vi "HP 6643A - GPIB Control.vi"() -> ()   [LabVIEW 2018]
doc: "This example performs a serial port write and a serial port read. The parameters set for the serial port must match the parameters of the connected instrument or device. The VISA Configure Serial Port VI sets the configuration parameters. The front panel displays the controls used to configure the basic parameters, such as baud rate, data bits, and parity. The VI passes the VISA resource name to other VIs that perform operations on that VISA resource. The VISA Write function sends a command to the serial device and the VISA Read function returns data based on the command. The VISA Close function then closes the reference to the serial device. It is important to close the reference; otherwise, further communication through that port might not be possible."
uses:
  <vilib>/Instr/_visa.llb/VISA Open Access Mode.ctl
panel:
  in  "Numeric":sgl format="%#.3f"
  out "Current (Amps)":dbl format="%.2f"
  out "Voltage (Volts)":dbl format="%.2f"
  in  "Output":bool
  out "Iterations":i32
  in  "stop":bool
  out "NewVal":dbl
  out "OldVal":dbl
  out "String":string
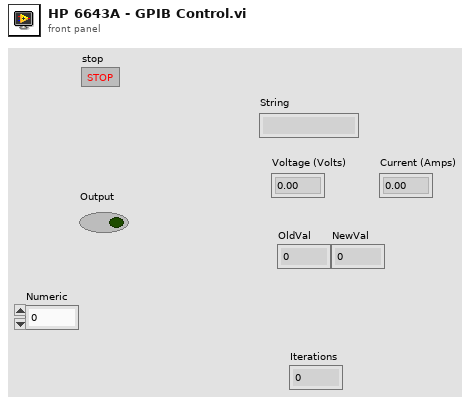
[diagram p1: front panel]
types:
  T1 = typedef "VISA Open Access Mode.ctl" = u32
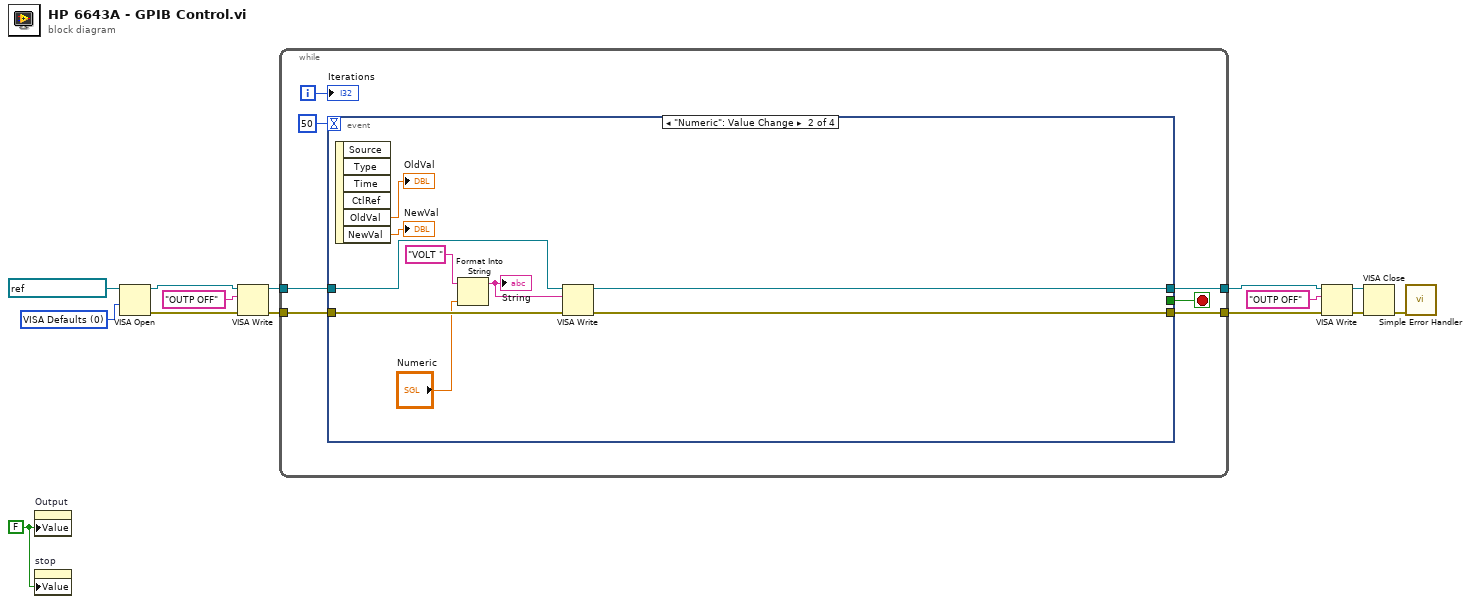
[diagram p0: block diagram]
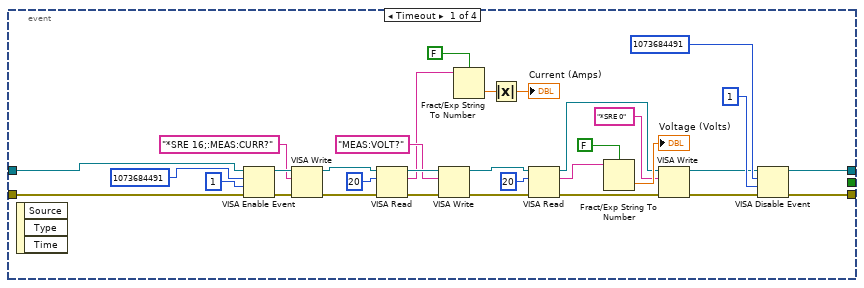
[diagram p2: hidden frame]
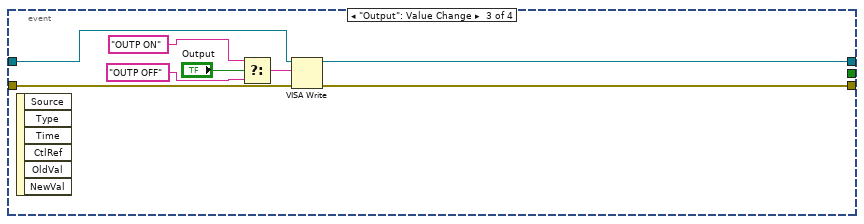
[diagram p3: hidden frame]
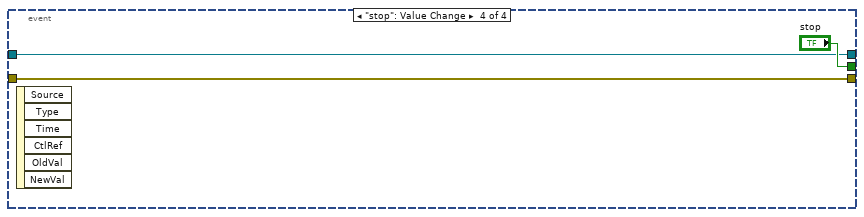
[diagram p4: hidden frame]
diagram:
  w2 = FALSE ("stop")
  w13 = T1 0 items=["VISA Defaults"=0, "Exclusive Lock"=1, "Load Configured Settings"=4] ("Access Mode")
  n1 = property on="Output" class="Bool (strict)"("Value"=w2) -> ()  [unwired: 2 in, 2 out]
  n2 = property on="stop" class="Bool (strict)"("Value"=w2) -> ()  [unwired: 2 in, 2 out]
  n3 = VISA Open(access mode=w13, VISA resource name=refnum<visa-resource-name> "DESK-06643A") -> (VISA resource name=w6:refnum<visa-resource-name>, error out=w7:errorcluster)  [unwired: 3 in]
  n4 = VISA Write(VISA resource name=w6, write buffer="OUTP OFF", error in (no error)=w7) -> (VISA resource name out=w4:refnum<visa-resource-name>, error out=w3:errorcluster)  [unwired: 1 out]
  n5 = while {
    tunnel: w3 -> [w21]
    tunnel: w4 -> [w20]
    tunnel: [w18] -> w10
    tunnel: [w19] -> w12
    i -> [w16]
    stop <- w17 stop-if-true
    n6 = event shown="[1] \"Numeric\": Value Change" {
      selector: _ -> [_ _ _ _]
      dyn-events: _ -> [_ _ _ _]
      timeout: 50 -> [_ _ _ _]
      tunnel: w21 -> [w25 w59 w69 w71]
      tunnel: w20 -> [w26 w60 w70 w72]
      tunnel: [w23 w58 w68 w71] -> w19
      tunnel: [w24 w57 w67 w72] -> w18
      tunnel: [_ _ _ "stop"] -> w17
      event Timeout {
        n7 = event-data() -> ()  [unwired: 1 in, 3 out]
        n8 = VISA Enable Event(8:w25, 9:u16 1, 10:u32 1073684491, 11:w26) -> (0:w38:errorcluster, 3:w39:refnum<visa-resource-name>)
        n9 = VISA Write(VISA resource name=w39, write buffer="*SRE 16;:MEAS:CURR?", error in (no error)=w38) -> (VISA resource name out=w30:refnum<visa-resource-name>, error out=w29:errorcluster)  [unwired: 1 out]
        n10 = VISA Read(VISA resource name=w30, byte count=20, error in (no error)=w29) -> (VISA resource name out=w52:refnum<visa-resource-name>, read buffer=w48:string, error out=w51:errorcluster)  [unwired: 1 out]
        n11 = VISA Write(VISA resource name=w52, write buffer="MEAS:VOLT?", error in (no error)=w51) -> (VISA resource name out=w28:refnum<visa-resource-name>, error out=w27:errorcluster)  [unwired: 1 out]
        n12 = Fract/Exp String To Number(use system decimal point (T)=FALSE, string=w48) -> (number=w46:dbl)  [unwired: 2 in, 1 out]
        n13 = Absolute Value(x=w46) -> (abs(x)=→"Current (Amps)":dbl)
        n14 = VISA Read(VISA resource name=w28, byte count=u32 20, error in (no error)=w27) -> (VISA resource name out=w43:refnum<visa-resource-name>, read buffer=w47:string, error out=w42:errorcluster)  [unwired: 1 out]
        n15 = Fract/Exp String To Number(use system decimal point (T)=FALSE, string=w47) -> (number=→"Voltage (Volts)":dbl)  [unwired: 2 in, 1 out]
        n16 = VISA Write(VISA resource name=w43, write buffer="*SRE 0", error in (no error)=w42) -> (VISA resource name out=w33:refnum<visa-resource-name>, error out=w34:errorcluster)  [unwired: 1 out]
        n17 = VISA Disable Event(8:w34, 9:u16 1, 10:u32 1073684491, 11:w33) -> (0:w23:errorcluster, 3:w24:refnum<visa-resource-name>)
      }
      event "Numeric": Value Change {
        n18 = event-data() -> ("OldVal"=→"OldVal":sgl, "NewVal"=→"NewVal":sgl)  [unwired: 1 in, 4 out]
        n19 = Format Into String(initial string="VOLT ", "Numeric") -> (resulting string=w62:string)  [unwired: 2 in, 1 out]
        "String" <- w62
        n20 = VISA Write(VISA resource name=w60, write buffer=w62, error in (no error)=w59) -> (VISA resource name out=w57:refnum<visa-resource-name>, error out=w58:errorcluster)  [unwired: 1 out]
      }
      event "Output": Value Change {
        n21 = event-data() -> ()  [unwired: 1 in, 6 out]
        n22 = Select(t="OUTP ON", s="Output", f="OUTP OFF") -> (s? t:f=w63:string)
        n23 = VISA Write(VISA resource name=w70, write buffer=w63, error in (no error)=w69) -> (VISA resource name out=w67:refnum<visa-resource-name>, error out=w68:errorcluster)  [unwired: 1 out]
      }
      event "stop": Value Change {
        n24 = event-data() -> ()  [unwired: 1 in, 6 out]
      }
    }
    "Iterations" <- w16
  }
  n25 = VISA Write(VISA resource name=w10, write buffer="OUTP OFF", error in (no error)=w12) -> (VISA resource name out=w9:refnum<visa-resource-name>, error out=w11:errorcluster)  [unwired: 1 out]
  n26 = VISA Close(VISA resource name=w9, error in (no error)=w11) -> (error out=w14:errorcluster)
  n27 = call <vilib>:"Simple Error Handler.vi"("error in (no error)"=w14) -> ()  [unwired: 1 in, 8 out]
